vi "Copy State Callbacks.vi"(7 "From":refnum<class "Endpoint.lvclass">, 8 "error in (no error)":errorcluster, 11 "Endpoint in":refnum<class "Endpoint.lvclass">) -> (0 "error out":errorcluster, 3 "Endpoint out":refnum<class "Endpoint.lvclass">)   [LabVIEW 2020, in "Stream.lvlib" / "Endpoint.lvclass"]
uses:
  Endpoint.lvclass
  Endpoint.lvclass/Endpoint.ctl
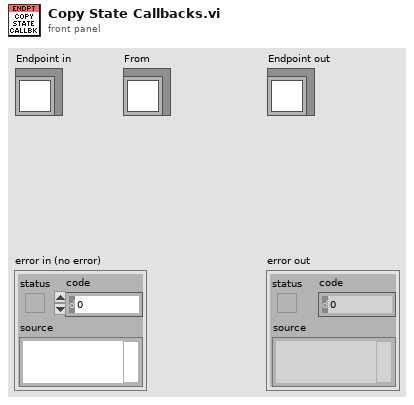
[diagram p1: front panel]
types:
  T1 = typedef "Stream.lvlib/Endpoint.lvclass/State Callback.ctl" = cluster{"Owner":refnum<class>, "VI":refnum<vi>}
  T2 = typedef "Stream.lvlib/Endpoint.lvclass/Ref Data.ctl" = cluster{"URI":refnum<class "URI.lvclass">, "State Callbacks":T1[], "Open":bool, "Mode":T3}
  T3 = typedef "Stream.lvlib/Mode.ctl" = enum16{"Raw", "Buffered", "LineTerm"}
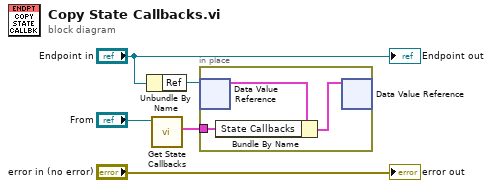
[diagram p0: block diagram]
diagram:
  n1 = Unbundle By Name("Endpoint in") -> ("Ref"=w3:refnum<data-value>)
  n2 = call "Get State Callbacks.vi"("Endpoint in"="From") -> ("State Callbacks"=w1:T1[])  [unwired: 8 in, 2 out]
  n3 = in-place {
    in-place-border: w1 -> [w6]
    n4 = in-place-dvr #1(w3) -> (w8:T2)  [unwired: 1 out]
    n5 = Bundle By Name(cluster=w8, "State Callbacks"=w6) -> (w7:T2)
    n6 = in-place-dvr #1(w7) -> ()  [unwired: 2 out]
  }
  "error out" <- "error in (no error)"
  "Endpoint out" <- "Endpoint in"
